vi "IO状态读取 (子VI).vi"(10 "传感器型号:":enum16{"PLC", "ZLAN", "ART"}(ring), 11 "端口:":T1(ring)) -> (3 "布尔":bool)   [LabVIEW 2016, in "环境动力监测库.lvlib"]
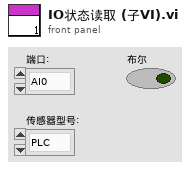
[diagram p1: front panel]
types:
  T1 = enum16{"AI0", "AI1", "AI2", "AI3", "AI4", "DI0", "DI1", "DI2", "DI3", "DI4", "DI5", "DI6", "DI7", "DO0", "DO1", "DO2", "DO3", "DO4", "DO5", "DO6", "DO7", "X0", "X1", "X2", "X3", "X4", "X5", "X6", "X7", "X8", "X9", "X10", "X11", "X12", "X13", "X14", "X15", "X16", "X17", "X18", "X19", "X20", "X21", "X22", "X23"}
  T2 = cluster{"状态":cluster{"R0":i16, "R1":i16, "R2":i16, "R3":i16, "R4":i16, "R5":i16, "R6":i16, "R7":i16, "R8":i16, "R9":i16, "R10":i16, "R11":i16, "R12":i16, "R13":i16, "R14":i16, "R15":i16, "R16":i16, "R17":i16, "R18":i16, "R19":i16, "R20":i16, "R21":i16, "R22":i16, "R23":i16, "R24":i16, "R25":i16, "R26":i16, "R27":i16, "R28":i16, "R29":i16, "R30":i16, "R31":i16, "R32":i16, "R33":i16, "R34":i16, "R35":i16, "R36":i16, "R37":i16, "R38":i16, "R39":i16}, "输入状态":bool[], "输出状态":bool[], "参数设置":cluster{"R100":i16, "R101":i16, "R102":i16, "R103":i16, "R104":i16, "R105":i16, "R106":i16, "R107":i16, "R108":i16, "R109":i16, "R110":i16, "R111":i16, "R112":i16, "R113":i16, "R114":i16, "R115":i16, "R116":i16, "R117":i16, "R118":i16, "R119":i16, "R120":i16, "R121":i16, "R122":i16, "R123":i16}, "转换值":cluster{"AD0":sgl, "AD1":sgl, "AD2":sgl, "AD3":sgl, "AD4":sgl, "AD5":sgl}}
  T3 = typedef "采配水类型.ctl" = enum16{"V1", "V2", "V3", "V4", "室内V1", "室内V2", "固定站V1", "固定站V2", "浮船V1", "浮船V2", "养殖尾水", "广东华南所"}
  T4 = cluster{"状态":cluster{"R0":i16, "R1":i16, "R2":i16, "R3":i16, "R4":i16, "R5":i16, "R6":i16, "R7":i16, "R8":i16, "R9":i16, "R10":i16, "R11":i16, "R12":i16, "R13":i16, "R14":i16, "R15":i16, "R16":i16, "R17":i16, "R18":i16, "R19":i16, "R20":i16, "R21":i16, "R22":i16, "R23":i16, "R24":i16, "R25":i16, "R26":i16, "R27":i16, "R28":i16, "R29":i16, "R30":i16, "R31":i16, "R32":i16, "R33":i16, "R34":i16, "R35":i16, "R36":i16, "R37":i16, "R38":i16, "R39":i16, "R40":i16, "R41":i16, "R42":i16, "R43":i16, "R44":i16, "R45":i16, "R46":i16, "R47":i16, "R48":i16, "R49":i16, "R50":i16, "R51":i16, "R52":i16, "R53":i16, "R54":i16, "R55":i16, "R56":i16, "R57":i16, "R58":i16, "R59":i16, "R60":i16, "R61":i16, "R62":i16, "R63":i16, "R64":i16, "R65":i16, "R66":i16, "R67":i16, "R68":i16, "R69":i16}, "输入状态":bool[], "输出状态":bool[], "报警簇":bool[], "参数设置":cluster{"R100":i16, "R101":i16, "R102":i16, "R103":i16, "R104":i16, "R105":i16, "R106":i16, "R107":i16, "R108":i16, "R109":i16, "R110":i16, "R111":i16, "R112":i16, "R113":i16, "R114":i16, "R115":i16, "R116":i16, "R117":i16, "R118":i16, "R119":i16, "R120":i16, "R121":i16, "R122":i16, "R123":i16, "R124":i16}, "转换值":cluster{"AD0":sgl, "AD1":sgl, "AD2":sgl, "AD3":sgl, "AD4":sgl, "AD5":sgl}, "看门狗启用":bool, "氨氮模块名称":string, "总磷模块名称":string, "采配水模块类型":T3}
  T5 = cluster{"环境变量":cluster{"蓄电池电压":dbl, "室温":dbl, "湿度":dbl, "水浸报警":bool, "烟雾报警":bool, "门禁1状态":bool, "门禁2状态":bool}, "ZLAN 6842 MB session":refnum<class "MB_Master.lvclass">, "DI":bool[], "DO":bool[]}
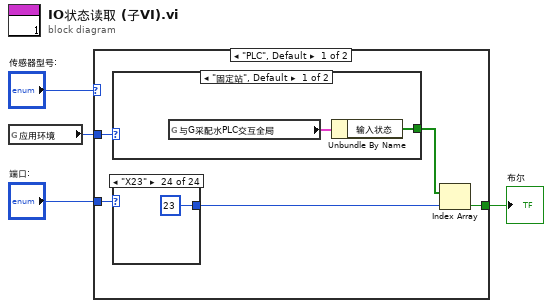
[diagram p0: block diagram]
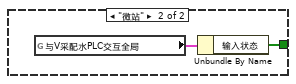
[diagram p2: hidden frame]
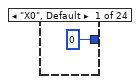
[diagram p3: hidden frame]
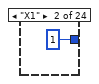
[diagram p4: hidden frame]
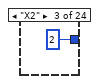
[diagram p5: hidden frame]
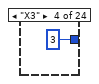
[diagram p6: hidden frame]
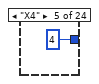
[diagram p7: hidden frame]
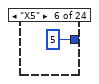
[diagram p8: hidden frame]
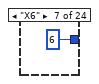
[diagram p9: hidden frame]
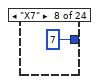
[diagram p10: hidden frame]
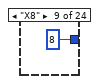
[diagram p11: hidden frame]
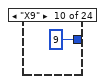
[diagram p12: hidden frame]
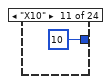
[diagram p13: hidden frame]
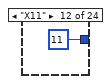
[diagram p14: hidden frame]
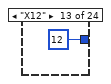
[diagram p15: hidden frame]
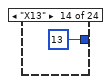
[diagram p16: hidden frame]
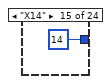
[diagram p17: hidden frame]
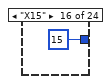
[diagram p18: hidden frame]
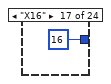
[diagram p19: hidden frame]
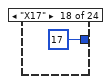
[diagram p20: hidden frame]
diagram:
  n1 = global read "外部交互全局变量.vi" "应用环境"() -> (w4:enum16{"固定站", "微站", "浮标", "浮船"})
  n2 = case shown="\"PLC\", Default" "传感器型号:" {
    tunnel: "端口:" -> [w9 w42]
    tunnel: [w7 w40] -> w3
    tunnel: w4 -> [w5 _]
    frame "PLC", Default {
      n3 = case shown="\"固定站\", Default" w5 {
        tunnel: [w10 w12] -> w6
        frame "固定站", Default {
          n4 = global read "外部交互全局变量.vi" "与G采配水PLC交互全局"() -> (w11:T2)
          n5 = Unbundle By Name(w11) -> ("输入状态"=w10:bool[])
        }
        frame "微站" {
          n6 = global read "外部交互全局变量.vi" "与V采配水PLC交互全局"() -> (w13:T4)
          n7 = Unbundle By Name(w13) -> ("输入状态"=w12:bool[])
        }
      }
      n8 = case shown="\"X23\"" w9 {
        tunnel: [0 ("索引") 1 ("索引") 2 ("索引") 3 ("索引") 4 ("索引") 5 ("索引") 6 ("索引") 7 ("索引") 8 ("索引") 9 ("索引") 10 ("索引") 11 ("索引") 12 ("索引") 13 ("索引") 14 ("索引") 15 ("索引") 16 ("索引") 17 ("索引") 18 ("索引") 19 ("索引") 20 ("索引") 21 ("索引") 22 ("索引") 23 ("索引")] -> w8
        frame "X0", Default {
        }
        frame "X1" {
        }
        frame "X2" {
        }
        frame "X3" {
        }
        frame "X4" {
        }
        frame "X5" {
        }
        frame "X6" {
        }
        frame "X7" {
        }
        frame "X8" {
        }
        frame "X9" {
        }
        frame "X10" {
        }
        frame "X11" {
        }
        frame "X12" {
        }
        frame "X13" {
        }
        frame "X14" {
        }
        frame "X15" {
        }
        frame "X16" {
        }
        frame "X17" {
        }
        frame "X18" {
        }
        frame "X19" {
        }
        frame "X20" {
        }
        frame "X21" {
        }
        frame "X22" {
        }
        frame "X23" {
        }
      }
      n9 = Index Array(array=w6, index=w8) -> (element=w7:bool)
    }
    frame "ZLAN" {
      n10 = global read "外部交互全局变量.vi" "与ZLAN交互全局"() -> (w39:T5)
      n11 = case shown="\"DI7\"" w42 {
        tunnel: [0 ("索引") 1 ("索引") 2 ("索引") 3 ("索引") 4 ("索引") 5 ("索引") 6 ("索引") 7 ("索引")] -> w41
        frame "DI0", Default {
        }
        frame "DI1" {
        }
        frame "DI2" {
        }
        frame "DI3" {
        }
        frame "DI4" {
        }
        frame "DI5" {
        }
        frame "DI6" {
        }
        frame "DI7" {
        }
      }
      n12 = Unbundle By Name(w39) -> ("DI"=w38:bool[])
      n13 = Index Array(array=w38, index=w41) -> (element=w40:bool)
    }
  }
  "布尔" <- w3
